vi "HeadingMod.vi"(1 "Heading":dbl) -> (0 "Heading Modified":dbl)   [LabVIEW 2014]
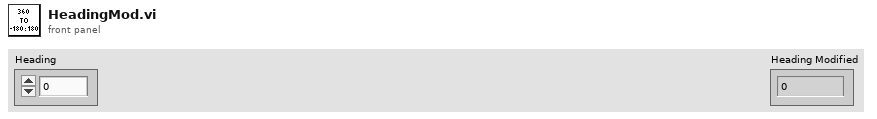
[diagram p1: front panel]
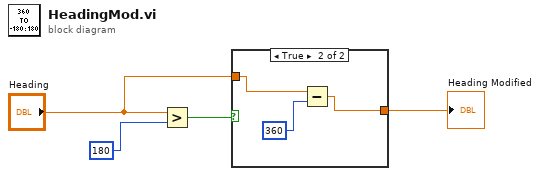
[diagram p0: block diagram]
diagram:
  n1 = Greater?(x="Heading", y=180) -> (0:w4:bool)
  n2 = case shown="True" w4 {
    tunnel: "Heading" -> [w5 w8]
    tunnel: [w5 w6] -> w1
    frame False {
    }
    frame True {
      n3 = Subtract(x=w8, y=360) -> (x-y=w6:dbl)
    }
  }
  "Heading Modified" <- w1
